vi "Example - Alignment (Basic).vi"() -> ()   [LabVIEW 2012]
doc: "This example shows how to use the UI Tools Alignment primitives to snap GObjects to the panel bounds."
panel:
  in  "Move":bool
  in  "Snap Band":i16=50 min=0 step=1
  # "Set to TRUE to have the \"Object\" follow the mouse cursor.\nSet to FALSE to have the \"Object\" stay in that position."
  # "Adjust the Snap Band parameter to determine the distance\nfrom the panel's sides where the \"Snap\" action will be activated."
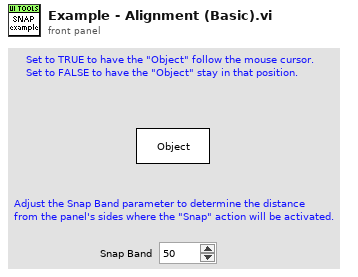
[diagram p1: front panel]
types:
  T1 = enum32{"invalid app kind", "Development System", "Run Time System", "Student Edition", "Embedded LabVIEW", "Evaluation", "Custom"}
  T2 = typedef "LVPoint32TypeDef.ctl" = cluster{"Horizontal":i32, "Vertical":i32}
  T3 = typedef "LVRectTypeDef.ctl" = cluster{"Left":i16, "Top":i16, "Right":i16, "Bottom":i16}
  T4 = cluster{"Left":i16, "Top":i16, "Left":i16, "Top":i16}
  T5 = cluster{"left":i16, "top":i16, "right":i16, "bottom":i16}
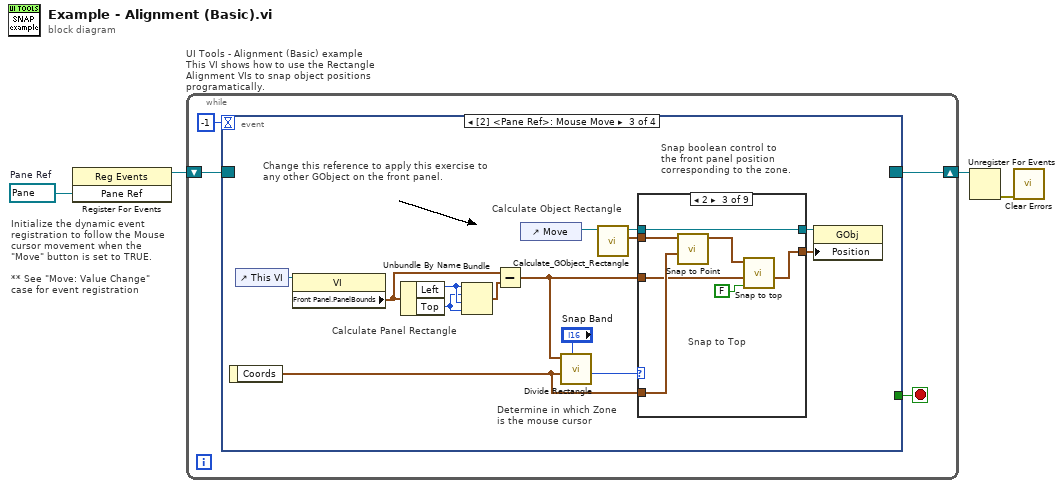
[diagram p0: block diagram]
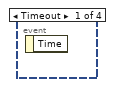
[diagram p2: hidden frame]
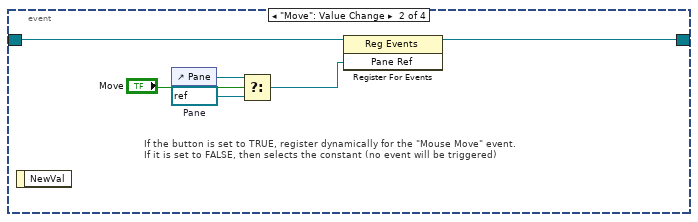
[diagram p3: hidden frame]
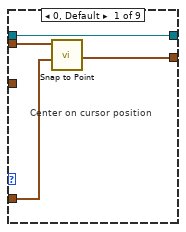
[diagram p4: hidden frame]
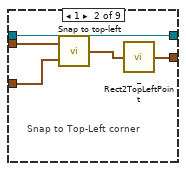
[diagram p5: hidden frame]
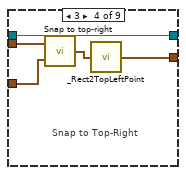
[diagram p6: hidden frame]
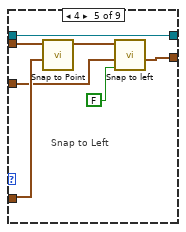
[diagram p7: hidden frame]
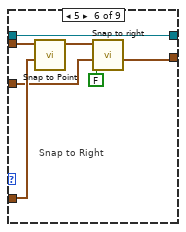
[diagram p8: hidden frame]
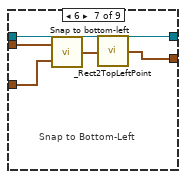
[diagram p9: hidden frame]
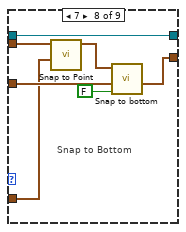
[diagram p10: hidden frame]
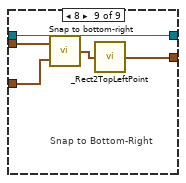
[diagram p11: hidden frame]
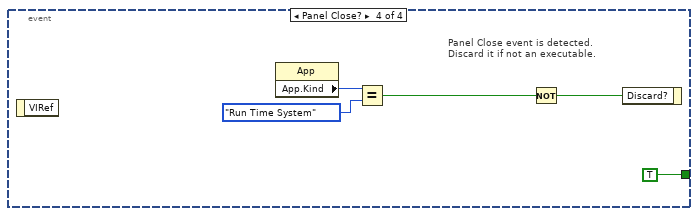
[diagram p12: hidden frame]
diagram:
  w3 = refnum<vi> refnum  # Pane Ref
  # "Initialize the dynamic event\nregistration to follow the Mouse\ncursor movement when the\n\"Move\" button is set to TRUE.\n\n** See \"Move: Value Change\"\ncase for event registration"
  n1 = register-events(w3) -> (reference out=w4:refnum<event-registration>)  [unwired: 2 in, 1 out]
  n2 = while "UI Tools - Alignment (Basic) example\nThis VI shows how to use the Rectangle Alignment VIs to snap object positions programatically." {
    shift-right: [w5] -> w1
    shift-left: w4 -> [w6]
    stop <- w7 stop-if-true
    n3 = event shown="[2] <Pane Ref>: Mouse Move" {
      selector: w6 -> [_ w12 _ _]
      dyn-events: [_ w10 _ _] -> w5
      timeout: -1 -> [_ _ _ _]
      tunnel: [_ _ _ TRUE ("Discard?")] -> w7
      event Timeout {
        n4 = event-data() -> ()  [unwired: 2 out]
      }
      event "Move": Value Change {
        w13 = refnum<vi> refnum  # Pane
        # "If the button is set to TRUE, register dynamically for the \"Mouse Move\" event.\nIf it is set to FALSE, then selects the constant (no event will be triggered)"
        n5 = event-data() -> ()  [unwired: 2 out]
        n6 = control-ref of="Pane"() -> (w14:refnum<vi>)
        n7 = Select(t=w14, s="Move", f=w13) -> (s? t:f=w11:refnum<vi>)
        n8 = register-events(reference=w12, w11) -> (reference out=w10:refnum<event-registration>)  [unwired: 1 in, 1 out]
      }
      event Mouse Move {
        # "Change this reference to apply this exercise to\nany other GObject on the front panel."
        # "Calculate Object Rectangle"
        # "Snap boolean control to\nthe front panel position\ncorresponding to the zone."
        # "Determine in which Zone\nis the mouse cursor"
        # "Calculate Panel Rectangle"
        n9 = event-data() -> ("Coords"=w23:T2)  [unwired: 1 out]
        n10 = control-ref of="This VI"() -> (w24:refnum<vi>)
        n11 = property class="VI"(reference=w24) -> ("Front Panel.PanelBounds"=w22:T3)  [unwired: 1 in, 2 out]
        n12 = Unbundle By Name(w22) -> ("Left"=w21:i16, "Top"=w20:i16)
        n13 = Bundle("Left"=w21, "Top"=w20, "Left"=w21, "Top"=w20) -> (w19:T4)  [unwired: 1 out]
        n14 = Subtract(x=w22, y=w19) -> (x-y=w18:T3)
        n15 = control-ref of="Move"() -> (w15:refnum<vi>)
        n16 = call "Divide Rectangle.vi"("Band (50)"="Snap Band", "Coords"=w23, "Rectangle"=w18) -> ("Zone"=w27:i32)  [unwired: 8 out]
        n17 = call "Calculate_GObject_Rectangle.vi"("GObject ref"=w15) -> ("Rectangle"=w25:T5, "GObject ref dup"=w17:refnum<vi>)  [unwired: 2 in, 7 out]
        n18 = case shown="2" w27 {
          tunnel: [w32 w35 w40 w49 w51 w59 w68 w74 w80] -> w26
          tunnel: w25 -> [w31 w33 w44 w48 w55 w62 w67 w73 w79]
          tunnel: w18 -> [_ w37 w42 w47 w52 w58 w66 w75 w78]
          tunnel: w23 -> [w30 _ w43 _ w54 w61 _ w71 _]
          tunnel: w17 -> [w29 w34 w38 w45 w56 w63 w64 w69 w76]
          tunnel: [w29 w34 w38 w45 w56 w63 w64 w69 w76] -> w16
          frame 0, Default {
            # "Center on cursor position"
            n19 = call "Snap to Point.vi"("Point"=w30, "Rect"=w31) -> ("TopLeft point"=w32:cluster{"x":i32, "y":i32})  [unwired: 9 out]
          }
          frame 1 {
            # "Snap to Top-Left corner"
            n20 = call "Snap to top-left.vi"("Fixed Rect"=w37, "Rect"=w33) -> ("Snapped to top left"=w36:T5)
            n21 = call "_Rect2TopLeftPoint.vi"("bounds"=w36) -> ("TopLeft point"=w35:cluster{"x":i32, "y":i32})  [unwired: 4 out]
          }
          frame 2 {
            # "Snap to Top"
            n22 = call "Snap to Point.vi"("Point"=w43, "Rect"=w44) -> ("Snapped to Point"=w41:T5)  [unwired: 9 out]
            n23 = call "Snap to top.vi"("centered? (F)"=FALSE, "Fixed Rect"=w42, "Rect"=w41) -> ("TopLeft point"=w40:cluster{"x":i32, "y":i32})  [unwired: 8 out]
          }
          frame 3 {
            # "Snap to Top-Right"
            n24 = call "Snap to top-right.vi"("Fixed Rect"=w47, "Rect"=w48) -> ("Snapped to top left"=w46:T5)
            n25 = call "_Rect2TopLeftPoint.vi"("bounds"=w46) -> ("TopLeft point"=w49:cluster{"x":i32, "y":i32})  [unwired: 4 out]
          }
          frame 4 {
            # "Snap to Left"
            n26 = call "Snap to Point.vi"("Point"=w54, "Rect"=w55) -> ("Snapped to Point"=w53:T5)  [unwired: 9 out]
            n27 = call "Snap to left.vi"("centered? (F)"=FALSE, "Fixed Rect"=w52, "Rect"=w53) -> ("TopLeft point"=w51:cluster{"x":i32, "y":i32})  [unwired: 8 out]
          }
          frame 5 {
            # "Snap to Right"
            n28 = call "Snap to Point.vi"("Point"=w61, "Rect"=w62) -> ("Snapped to Point"=w60:T5)  [unwired: 9 out]
            n29 = call "Snap to right.vi"("centered? (F)"=FALSE, "Fixed Rect"=w58, "Rect"=w60) -> ("TopLeft point"=w59:cluster{"x":i32, "y":i32})  [unwired: 8 out]
          }
          frame 6 {
            # "Snap to Bottom-Left"
            n30 = call "Snap to bottom-left.vi"("Fixed Rect"=w66, "Rect"=w67) -> ("Snapped to bottom left"=w65:T5)
            n31 = call "_Rect2TopLeftPoint.vi"("bounds"=w65) -> ("TopLeft point"=w68:cluster{"x":i32, "y":i32})  [unwired: 4 out]
          }
          frame 7 {
            # "Snap to Bottom"
            n32 = call "Snap to Point.vi"("Point"=w71, "Rect"=w73) -> ("Snapped to Point"=w72:T5)  [unwired: 9 out]
            n33 = call "Snap to bottom.vi"("centered? (F)"=FALSE, "Fixed Rect"=w75, "Rect"=w72) -> ("TopLeft point"=w74:cluster{"x":i32, "y":i32})  [unwired: 8 out]
          }
          frame 8 {
            # "Snap to Bottom-Right"
            n34 = call "Snap to bottom-right.vi"("Fixed Rect"=w78, "Rect"=w79) -> ("Snapped to bottom right"=w77:T5)
            n35 = call "_Rect2TopLeftPoint.vi"("bounds"=w77) -> ("TopLeft point"=w80:cluster{"x":i32, "y":i32})  [unwired: 4 out]
          }
        }
        n36 = property class="GObj"(reference=w16, "Position"=w26) -> ()  [unwired: 1 in, 2 out]
      }
      event Panel Close? {
        # "Panel Close event is detected.\nDiscard it if not an executable."
        n37 = event-data() -> ()  [unwired: 2 out]
        n38 = property class="App"() -> ("App.Kind"=w84:T1)  [unwired: 2 in, 2 out]
        n39 = Equal?(x=w84, y=T1."Run Time System" ("Application:Kind")) -> (x = y?=w83:bool)
        n40 = Not(x=w83) -> (.not. x?=w81:bool)
        n41 = event-data("Discard?"=w81) -> ()  [unwired: 1 in, 1 out]
      }
    }
  }
  n42 = Unregister For Events(event registration refnum=w1) -> (error out=w2:errorcluster)  [unwired: 1 in]
  n43 = call <vilib>:"Clear Errors.vi"("error in (no error)"=w2) -> ()  [unwired: 7 out]
